vi "Get Value.vi"(8 "error in":errorcluster, 10 "Key":string, 11 "Section in":refnum<class "Section.lvclass">) -> (0 "error out":errorcluster, 1 "Value":refnum<class "Value.lvclass">, 2 "Found?":bool, 3 "Section out":refnum<class "Section.lvclass">)   [LabVIEW 2019, in "Electronic Datasheet.lvlib" / "Section.lvclass"]
uses:
  Section.lvclass
  Value/Value.lvclass
  Section.lvclass/Section.ctl
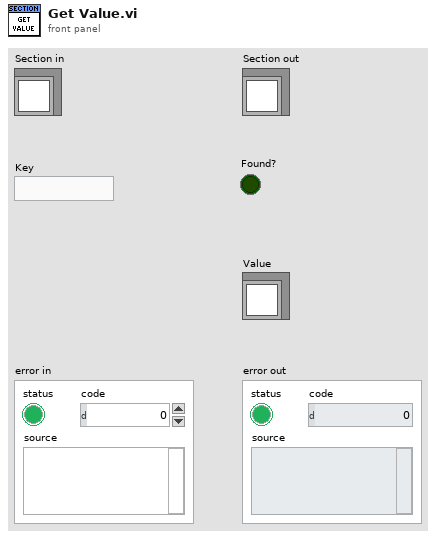
[diagram p1: front panel]
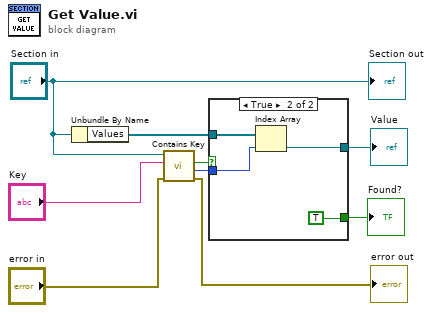
[diagram p0: block diagram]
diagram:
  n1 = Unbundle By Name("Section in") -> ("Values"=w9:refnum<class "Value.lvclass">[])
  n2 = call "Contains Key.vi"("error in"="error in", "Key"="Key", "Section in"="Section in") -> ("error out"=→"error out":errorcluster, "Index"=w1:i32, "Contains Key?"=w5:bool)  [unwired: 5 in, 1 out]
  n3 = case shown="True" w5 {
    selector: w5 -> [w10 _]
    tunnel: w9 -> [_ w14]
    tunnel: [_ w13] -> w4
    tunnel: [w10 TRUE] -> w8
    tunnel: w1 -> [_ w11]
    frame False {
    }
    frame True {
      n4 = Index Array(array=w14, index=w11) -> (element=w13:refnum<class "Value.lvclass">)
    }
  }
  "Found?" <- w8
  "Value" <- w4
  "Section out" <- "Section in"
